vi "write_data.vi"(8 "error in (no error)":errorcluster, 10 "data":T1, 11 "LatentDirichletAllocation in":refnum<class "LatentDirichletAllocation.lvclass">) -> (0 "error out":errorcluster, 3 "LatentDirichletAllocation out":refnum<class "LatentDirichletAllocation.lvclass">)   [LabVIEW 2020, in "LatentDirichletAllocation.lvclass"]
uses:
  LatentDirichletAllocation.lvclass
  Controls/latent_dirichlet_allocation_data.ctl
  LatentDirichletAllocation.lvclass/LatentDirichletAllocation.ctl
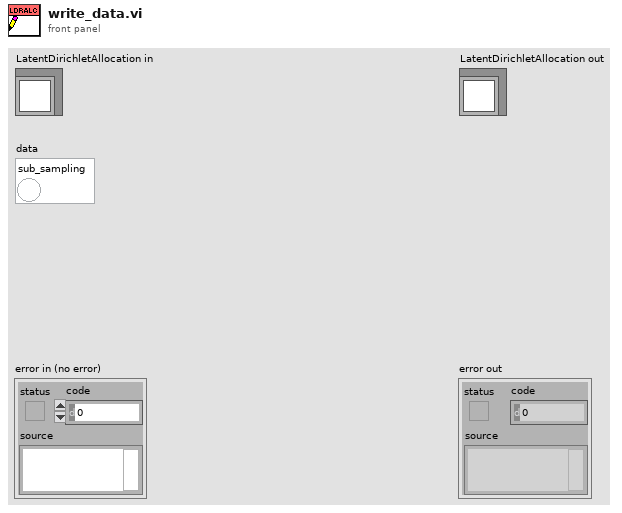
[diagram p1: front panel]
types:
  T1 = typedef "latent_dirichlet_allocation_data.ctl" = cluster{"sub_sampling":bool}
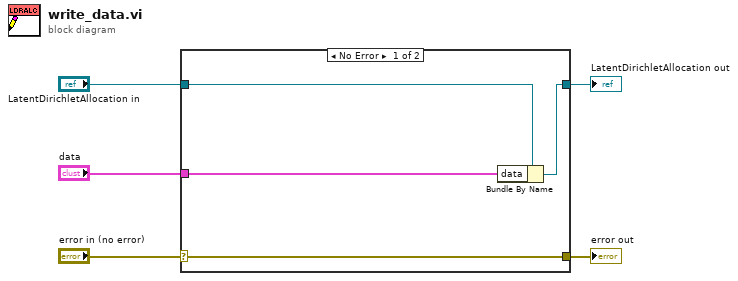
[diagram p0: block diagram]
diagram:
  n1 = case shown="No Error" "error in (no error)" {
    selector: "error in (no error)" -> [w9 w10]
    tunnel: [w9 w10] -> w4
    tunnel: [w7 w11] -> w2
    tunnel: "LatentDirichletAllocation in" -> [w8 w11]
    tunnel: "data" -> [w6 _]
    frame No Error {
      n2 = Bundle By Name(cluster=w8, "data"=w6) -> (w7:refnum<class "LatentDirichletAllocation.lvclass">)
    }
    frame Error {
    }
  }
  "error out" <- w4
  "LatentDirichletAllocation out" <- w2
